vi "REVISA_ARCHIVO.vi"(8 "error in (no error)":errorcluster, 11 "Conection path":path) -> (0 "error out":errorcluster, 3 "Conection path DUP":path)   [LabVIEW 2019, in "DB_VENDING MACHINE.lvlib"]
uses:
  DB_VENDING MACHINE.lvlib
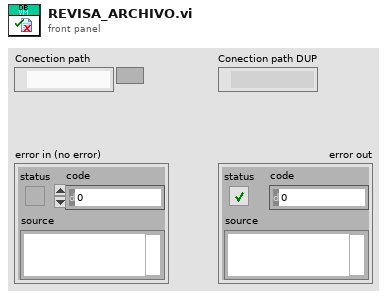
[diagram p1: front panel]
types:
  T1 = enum16{"open", "replace", "create", "open or create", "replace or create", "replace or create with confirmation"}
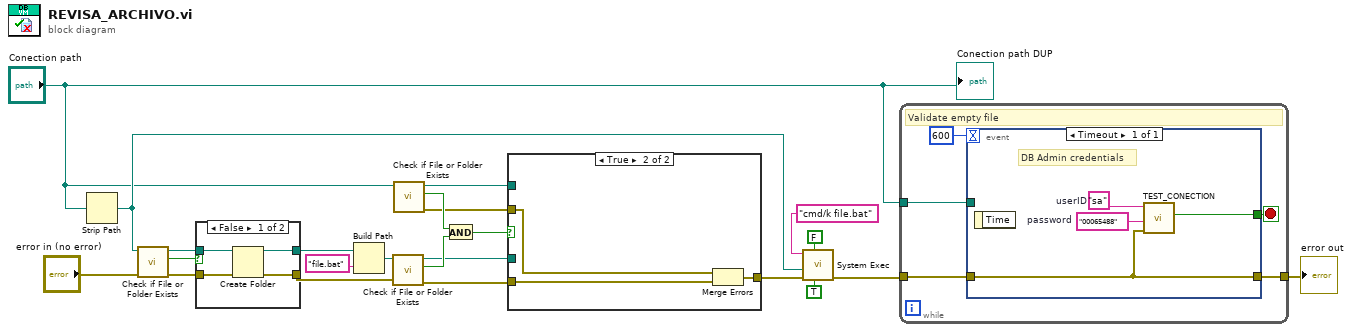
[diagram p0: block diagram]
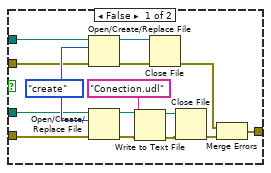
[diagram p2: hidden frame]
diagram:
  n1 = Strip Path(path="Conection path") -> (stripped path=w7:path)  [unwired: 1 out]
  n2 = call <vilib>:"Check if File or Folder Exists.vi"("error in (no error)"="error in (no error)", "path"=w7) -> ("error out"=w22:errorcluster, "file or folder exists?"=w23:bool, "dup path"=w21:path)  [unwired: 7 in]
  n3 = case shown="False" w23 {
    tunnel: w22 -> [w25 w28]
    tunnel: w21 -> [w27 w29]
    tunnel: [w26 w29] -> w19
    tunnel: [w24 w28] -> w16
    frame False {
      n4 = Create Folder(path (use dialog)=w27, error in=w25) -> (created path=w26:path, error out=w24:errorcluster)  [unwired: 1 in, 1 out]
    }
    frame True {
    }
  }
  n5 = Build Path(base path=w19, name or relative path="file.bat") -> (appended path=w17:path)
  n6 = call <vilib>:"Check if File or Folder Exists.vi"("error in (no error)"=w16, "path"=w17) -> ("error out"=w9:errorcluster, "file or folder exists?"=w14:bool, "dup path"=w10:path)  [unwired: 7 in]
  n7 = call <vilib>:"Check if File or Folder Exists.vi"("path"="Conection path") -> ("error out"=w11:errorcluster, "file or folder exists?"=w15:bool, "dup path"=w12:path)  [unwired: 8 in]
  n8 = And(x=w15, y=w14) -> (x .and. y?=w13:bool)
  n9 = case shown="True" w13 {
    tunnel: w12 -> [w41 _]
    tunnel: w11 -> [w40 w46]
    tunnel: w10 -> [w39 _]
    tunnel: w9 -> [w38 w47]
    tunnel: [w30 w45] -> w8
    frame False {
      w42 = T1."create" ("operation (0:open)")
      n10 = Open/Create/Replace File(file path (use dialog)=w41, error in=w40, operation (0:open)=w42) -> (refnum out=w43:refnum<file>, error out=w44:errorcluster)  [unwired: 3 in, 1 out]
      n11 = Open/Create/Replace File(file path (use dialog)=w39, error in=w38, operation (0:open)=w42) -> (refnum out=w37:refnum<file>, error out=w36:errorcluster)  [unwired: 3 in, 1 out]
      n12 = Write to Text File(file (use dialog)=w37, text="Conection.udl", error in=w36) -> (refnum out=w34:refnum<file>, error out=w35:errorcluster)  [unwired: 1 in, 1 out]
      n13 = Close File(refnum=w43, error in=w44) -> (error out=w31:errorcluster)  [unwired: 1 out]
      n14 = Close File(refnum=w34, error in=w35) -> (error out=w32:errorcluster)  [unwired: 1 out]
      n15 = Merge Errors(w31, w32) -> (w30:errorcluster)
    }
    frame True {
      n16 = Merge Errors(w46, w47) -> (w45:errorcluster)
    }
  }
  n17 = call <vilib>:"System Exec.vi"("run minimized? (F)"=TRUE, "wait until completion? (T)"=FALSE, "error in (no error)"=w8, "working directory"=w7, "command line"="cmd/k file.bat") -> ("error out"=w3:errorcluster)  [unwired: 3 in, 3 out]
  n18 = while {
    tunnel: w3 -> [w49]
    tunnel: "Conection path" -> [w51]
    tunnel: [w48] -> w1
    stop <- w50 stop-if-true
    # "Validate empty file"
    n19 = event shown="[0] Timeout" {
      selector: _ -> [_]
      dyn-events: _ -> [_]
      timeout: 600 -> [_]
      tunnel: w51 -> [_]
      tunnel: [w56] -> w50
      tunnel: w49 -> [w55]
      tunnel: [w55] -> w48
      event Timeout {
        w54 = "00065488"  # password
        w53 = "sa"  # userID
        # "DB Admin credentials"
        n20 = event-data() -> ()  [unwired: 1 in, 1 out]
        n21 = call "TEST_CONECTION.vi"("error in (no error)"=w55, "password"=w54, "userID"=w53) -> ("Test Connection"=w56:bool)  [unwired: 8 in]
      }
    }
  }
  "error out" <- w1
  "Conection path DUP" <- "Conection path"
